vi "Read Configuration Version v2.vi"(8 "error in (no error)":errorcluster, 11 "Configuration Session in":refnum<class "Configuration Session.lvclass">) -> (0 "error out":errorcluster, 2 "version":T1, 3 "Configuration Session out":refnum<class "Configuration Session.lvclass">)   [LabVIEW 2017, in "DSF Configuration.lvlib" / "Configuration Session.lvclass"]
uses:
  Configuration Session.lvclass
  DSF Configuration API/Public/Controls/DSF Version Info.ctl
  Configuration Session.lvclass/Configuration Session.ctl
  DSF Configuration.lvlib
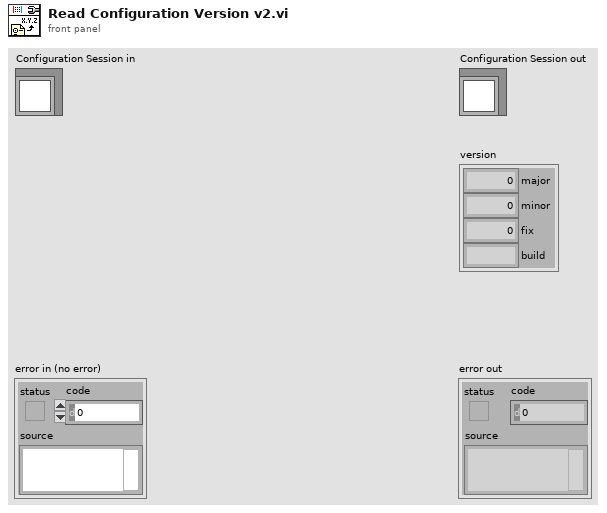
[diagram p1: front panel]
types:
  T1 = typedef "DSF Configuration.lvlib/DSF Version Info.ctl" = cluster{"major":u32, "minor":u32, "fix":u32, "build":string}
  T2 = typedef "DSF Configuration.lvlib/Configuration Session.lvclass/Config Data Ref.ctl" = refnum<data-value>
  T3 = typedef "DSF Configuration.lvlib/DSF Config Data.ctl" = cluster{"dsf configuration":T4, "path":path, "dirty":bool}
  T4 = typedef "DSF Configuration.lvlib/Internal.DSF Configuration.ctl" = cluster{"dsfversion":T1, "version":T1, "plugins":T5[], "groups":T8[], "transfers":T10[], "channels":T12[], "settings":T14[]}
  T5 = typedef "DSF Configuration.lvlib/Internal.DSF Plugin with ID.ctl" = cluster{"id":string, "values":T6}
  T6 = typedef "DSF Configuration.lvlib/Internal.DSF Plugin Info.ctl" = cluster{"type":string, "timing":T7, "group ids":string[], "settings id":string}
  T7 = typedef "DSF Configuration.lvlib/DSF Timing Info.ctl" = cluster{"priority":u64, "decimation":u64, "offset":u64}
  T8 = typedef "DSF Configuration.lvlib/Internal.DSF Group with ID.ctl" = cluster{"id":string, "values":T9}
  T9 = typedef "DSF Configuration.lvlib/Internal.DSF Group Info.ctl" = cluster{"direction":i32, "timing":T7, "transfer ids":string[], "settings id":string}
  T10 = typedef "DSF Configuration.lvlib/Internal.DSF Transfer with ID.ctl" = cluster{"id":string, "values":T11}
  T11 = typedef "DSF Configuration.lvlib/Internal.DSF Transfer Info.ctl" = cluster{"byte order":i32, "channel ids":string[], "settings id":string}
  T12 = typedef "DSF Configuration.lvlib/Internal.DSF Channel with ID.ctl" = cluster{"id":string, "values":T13}
  T13 = typedef "DSF Configuration.lvlib/Internal.DSF Channel Info.ctl" = cluster{"count":u64, "buffer offset":u64, "data type":i32, "settings id":string}
  T14 = typedef "DSF Configuration.lvlib/Internal.DSF Settings with ID.ctl" = cluster{"id":string, "values":T15}
  T15 = typedef "DSF Configuration.lvlib/Internal.DSF Settings Info.ctl" = cluster{"key":string, "value":string}[]
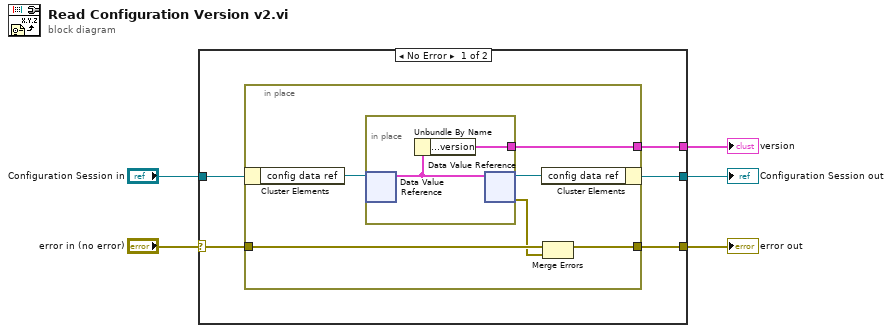
[diagram p0: block diagram]
diagram:
  n1 = case shown="No Error" "error in (no error)" {
    selector: "error in (no error)" -> [w7 w20]
    tunnel: [w6 w20] -> w4
    tunnel: "Configuration Session in" -> [w10 w19]
    tunnel: [w9 _] -> w1
    tunnel: [w8 w19] -> w2
    frame No Error {
      n2 = in-place {
        in-place-border: [w15] -> w9
        in-place-border: w7 -> [w13]
        in-place-border: [w11] -> w6
        n3 = in-place-cluster #1(w10) -> ("config data ref"=w16:T2)
        n4 = in-place {
          in-place-border: [w17] -> w15
          n5 = in-place-dvr #2(w16) -> (w18:T3)  [unwired: 1 out]
          n6 = Unbundle By Name(w18) -> ("dsf configuration.version"=w17:T1)
          n7 = in-place-dvr #2(w18) -> (w14:T2, w12:errorcluster)
        }
        n8 = in-place-cluster #1("config data ref"=w14) -> (w8:refnum<class "Configuration Session.lvclass">)
        n9 = Merge Errors(w13, w12) -> (w11:errorcluster)
      }
    }
    frame Error {
    }
  }
  "error out" <- w4
  "Configuration Session out" <- w2
  "version" <- w1
